vi "Evaluate Parent ID.vi"(11 "Linked List Definition in":refnum<class "Linked List Definition.lvclass">) -> (1 "Invalid Parent ID":bool, 2 "Parent ID":string, 3 "Linked List Definition out":refnum<class "Linked List Definition.lvclass">)   [LabVIEW 2020, in "Linked Lists.lvlib" / "Linked List Definition.lvclass"]
uses:
  <vilib>/gpm_packages/@cs/linked-list/Source/Linked List/Linked List Definition/Linked List Definition.lvclass
  <vilib>/gpm_packages/@cs/linked-list/Source/Linked List/Linked List Definition/Linked List Definition.lvclass/Linked List Definition.ctl
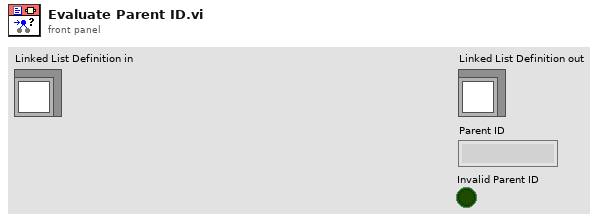
[diagram p1: front panel]
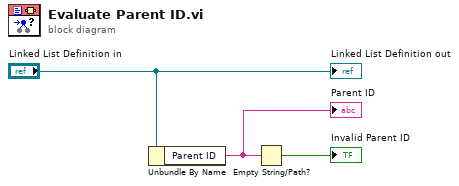
[diagram p0: block diagram]
diagram:
  n1 = Unbundle By Name("Linked List Definition in") -> ("Parent ID"=w2:string)
  "Parent ID" <- w2
  n2 = Empty String/Path?(string/path=w2) -> (empty?=→"Invalid Parent ID":bool)
  "Linked List Definition out" <- "Linked List Definition in"
